vi "pump_close.vi"(9 "error in (no error)":errorcluster, 11 "VISA resource name":refnum<visa-resource-name>) -> (1 "error out":errorcluster)   [LabVIEW 2020]
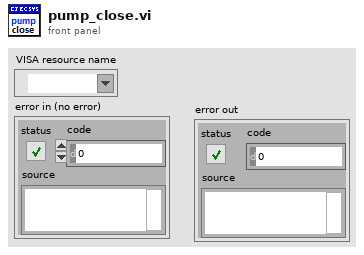
[diagram p1: front panel]
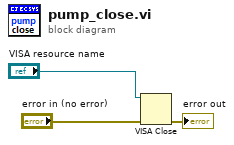
[diagram p0: block diagram]
diagram:
  n1 = VISA Close(VISA resource name="VISA resource name", error in (no error)="error in (no error)") -> (error out=→"error out":errorcluster)
